vi "OEE_SCREEN_2_generate_hourly_graph_values.vi"(11 "SCREEN_2_graph_hourly_all_info":T1={"hour_start"=8, "hour_end"=8, "actual_by_hour"=[], "target_by_hour"=[], "X_axis_labels"=[], "SCREEN_2_graph_hourly_references"={"graph_hourly"=refnum, "labels_picture_hourly"=refnum, "front_panel_reference"=refnum}}) -> (1 "Y_scale_max":dbl=160.0, 2 "Y_annotation_offset":dbl=7.9750000000000005, 3 "graph_values":cluster{dbl[], dbl[]}[](array[cluster])=[{[8.5, 9.5, 10.5, 11.5, 12.5, 13.5, 14.5, 15.5, 16.5, 17.5, 18.5, 19.5], [1.0, 5.0, 7.0, 0.0, 0.0, 0.0, 0.0, 0.0, 0.0, 0.0, 0.0, 0.0]}, {[8.5, 9.5, 10.5, 11.5, 12.5, 13.5, 14.5, 15.5, 16.5, 17.5, 18.5, 19.5], [10.0, 20.0, 30.0, 40.0, 50.0, 60.0, 70.0, 80.0, 90.0, 110.0, 120.0, 130.0]}])   [LabVIEW 2019]
uses:
  FGV/FGV_SCREEN_2_graph_hourly/FGV_SCREEN_2_graph_hourly_all_info.ctl
  FGV/FGV_SCREEN_2_graph_hourly/FGV_SCREEN_2_graph_hourly_references.ctl
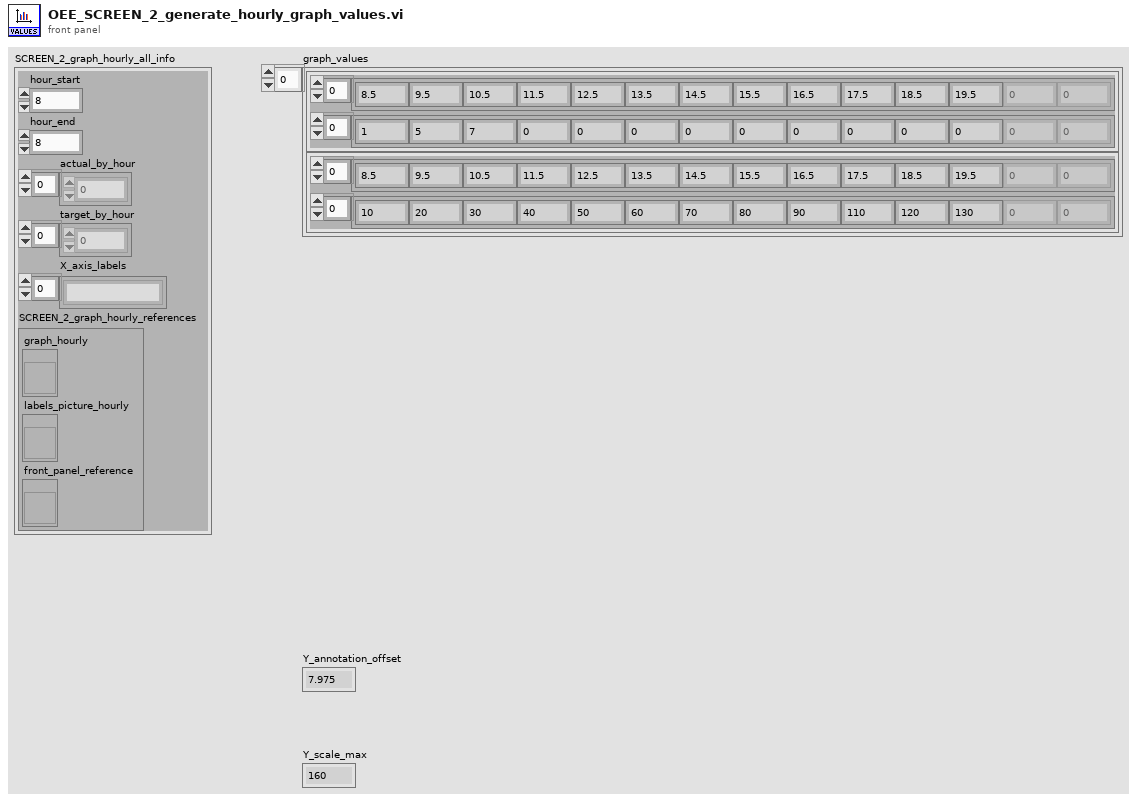
[diagram p1: front panel]
types:
  T1 = typedef "FGV_SCREEN_2_graph_hourly_all_info.ctl" = cluster{"hour_start":i8, "hour_end":i8, "actual_by_hour":u16[], "target_by_hour":u16[], "X_axis_labels":string[], "SCREEN_2_graph_hourly_references":T2}
  T2 = typedef "FGV_SCREEN_2_graph_hourly_references.ctl" = cluster{"graph_hourly":refnum<vi>, "labels_picture_hourly":refnum<vi>, "front_panel_reference":refnum<vi>}
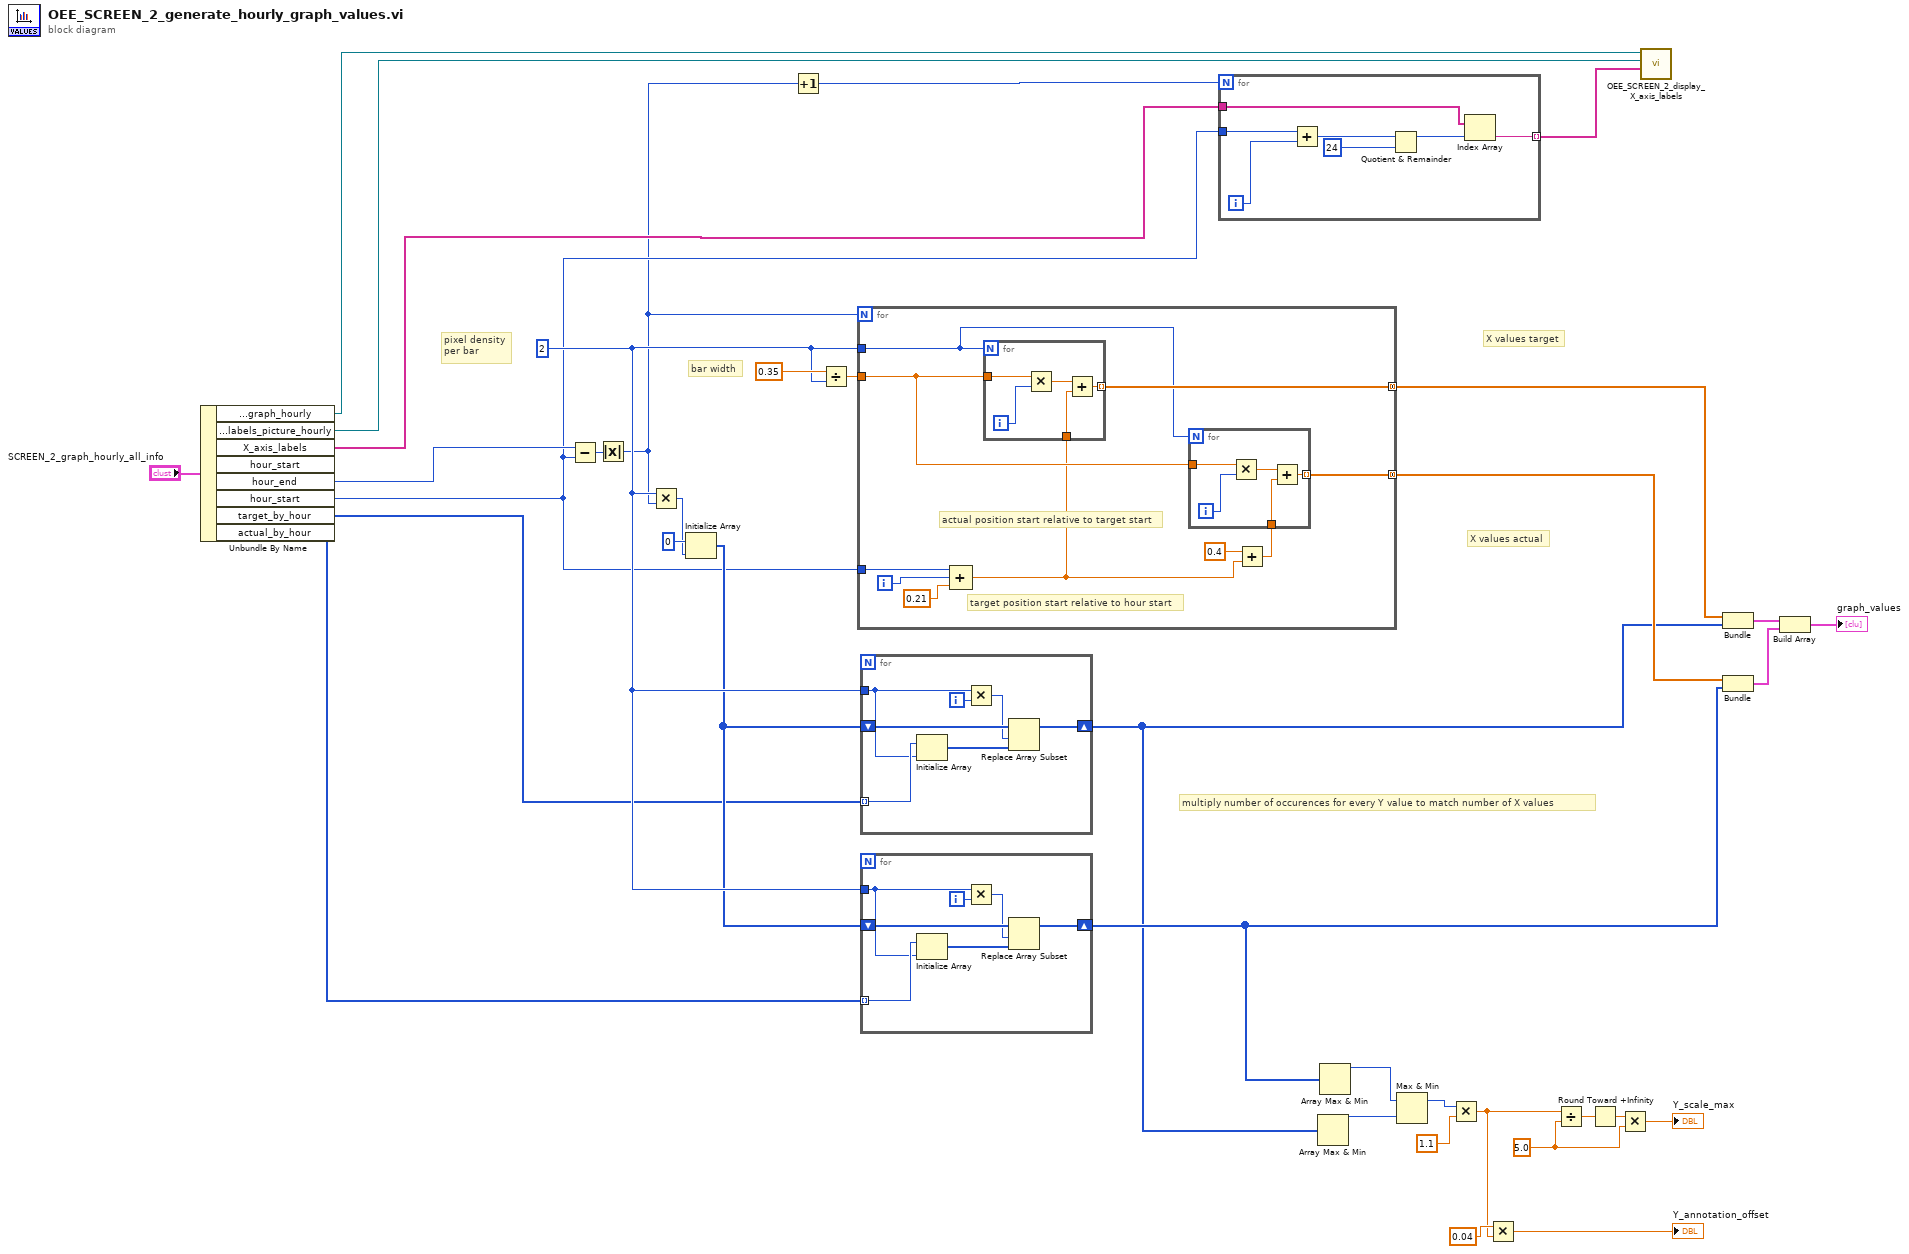
[diagram p0: block diagram]
diagram:
  w14 = 5.0 ("y")
  w21 = 2 ("x")
  # "multiply number of occurences for every Y value to match number of X values"
  # "X values target"
  # "X values actual"
  # "pixel density\nper bar"
  # "bar width"
  n1 = Unbundle By Name("SCREEN_2_graph_hourly_all_info") -> ("SCREEN_2_graph_hourly_references.graph_hourly"=w7:refnum<vi>, "SCREEN_2_graph_hourly_references.labels_picture_hourly"=w6:refnum<vi>, "X_axis_labels"=w4:string[], "hour_end"=w11:i8, "hour_start"=w3:i8, "target_by_hour"=w10:u16[], "actual_by_hour"=w9:u16[])  [unwired: 1 out]
  n2 = Subtract(x=w11, y=w3) -> (x-y=w2:i8)
  n3 = Absolute Value(x=w2) -> (abs(x)=w1:i8)
  n4 = Multiply(x=w21, y=w1) -> (x*y=w23:i32)
  n5 = Initialize Array(u16 0, w23) -> (w20:u16[])
  n6 = Increment(x=w1) -> (x+1=w5:i8)
  n7 = Divide(x=0.35, y=w21) -> (x/y=w25:dbl)
  n8 = for {
    N: w1 -> [_]
    tunnel: w3 -> [w46]
    tunnel: w21 -> [w37]
    tunnel: [w43] -> w22 mode=concatenating
    tunnel: w25 -> [w42]
    tunnel: [w38] -> w24 mode=concatenating
    i -> [w45]
    # "actual position start relative to target start"
    # "target position start relative to hour start"
    n9 = Compound Arithmetic op=unknown(w46, w45, 0.21 ("value")) -> (w41:dbl)
    n10 = for {
      N: w37 -> [_]
      tunnel: w41 -> [w54]
      tunnel: [w53] -> w43 mode=indexing
      tunnel: w42 -> [w52]
      i -> [w56]
      n11 = Multiply(x=w52, y=w56) -> (x*y=w55:dbl)
      n12 = Add(x=w55, y=w54) -> (x+y=w53:dbl)
    }
    n13 = Add(x=0.4, y=w41) -> (x+y=w39:dbl)
    n14 = for {
      N: w37 -> [_]
      tunnel: w39 -> [w49]
      tunnel: [w48] -> w38 mode=indexing
      tunnel: w42 -> [w47]
      i -> [w51]
      n15 = Multiply(x=w47, y=w51) -> (x*y=w50:dbl)
      n16 = Add(x=w50, y=w49) -> (x+y=w48:dbl)
    }
  }
  n17 = for {
    tunnel: w21 -> [w58]
    tunnel: w10 -> [w62] mode=indexing
    shift-right: [w57] -> w18
    shift-left: w20 -> [w63]
    i -> [w60]
    n18 = Initialize Array(w62, w58) -> (w61:u16[])
    n19 = Multiply(x=w58, y=w60) -> (x*y=w59:i32)
    n20 = Replace Array Subset(array=w63, new element=w61, index=w59) -> (w57:u16[])
  }
  n21 = for {
    tunnel: w21 -> [w65]
    tunnel: w9 -> [w69] mode=indexing
    shift-right: [w64] -> w19
    shift-left: w20 -> [w70]
    i -> [w67]
    n22 = Initialize Array(w69, w65) -> (w68:u16[])
    n23 = Multiply(x=w65, y=w67) -> (x*y=w66:i32)
    n24 = Replace Array Subset(array=w70, new element=w68, index=w66) -> (w64:u16[])
  }
  n25 = for {
    N: w5 -> [_]
    tunnel: w3 -> [w74]
    tunnel: w4 -> [w72]
    tunnel: [w71] -> w8 mode=indexing
    i -> [w73]
    n26 = Add(x=w74, y=w73) -> (x+y=w77:i32)
    n27 = Quotient & Remainder(x=w77, y=24) -> (x-y*floor(x/y)=w75:i32)  [unwired: 1 out]
    n28 = Index Array(array=w72, index=w75) -> (element=w71:string)
  }
  n29 = Array Max & Min(array=w18) -> (max value=w31:u16)  [unwired: 3 out]
  n30 = Array Max & Min(array=w19) -> (max value=w32:u16)  [unwired: 3 out]
  n31 = Max & Min(x=w32, y=w31) -> (max(x,y)=w30:u16)  [unwired: 1 out]
  n32 = Multiply(x=w30, y=1.1) -> (x*y=w17:dbl)
  n33 = Multiply(x=0.04 ("y"), y=w17) -> (x*y=→"Y_annotation_offset":dbl)
  n34 = Divide(x=w17, y=w14) -> (x/y=w16:dbl)
  n35 = Round Toward +Infinity(x=w16) -> (ceil(x): smallest int >= x=w15:dbl)
  n36 = Multiply(x=w15, y=w14) -> (x*y=→"Y_scale_max":dbl)
  n37 = call "OEE_SCREEN_2_display_X_axis_labels.vi"("labels"=w8, "labels_picture_accumulative"=w6, "XYGraph in"=w7) -> ()  [unwired: 9 in]
  n38 = Bundle(w22, w18) -> (w36:cluster{dbl[], u16[]})  [unwired: 1 in]
  n39 = Bundle(w24, w19) -> (w34:cluster{dbl[], u16[]})  [unwired: 1 in]
  n40 = Build Array(w36, w34) -> (→"graph_values":cluster{dbl[], u16[]}[])
